vi "Initalize (seq）(SubVI).vi"(10 "字符串":string, 11 "队列输入":refnum<queue>) -> ()   [LabVIEW 2019, in "Take Seq.lvlib"]
uses:
  Take Seq.lvlib
  config.ctl
  Instrument.ctl
  lib/QDInstrument.dll
  SubVI.lvlib
panel:
  # "(真是通道1，假是通道2)"
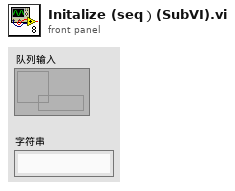
[diagram p1: front panel]
types:
  T1 = typedef "config.ctl" = cluster{"initialize":string, "6221":cluster{"6221 Resource":refnum<visa-resource-name>, "Delta status":bool}, "7001":cluster{"Ch":bool}, "SR830+6221":cluster{"source":u16, "阻抗":dbl, "量程入 4":i32, "量程入 3":i32, "量程入 2":i32, "量程入 1":i32, "电流":dbl, "SR830 2":bool, "SR830 3":bool, "SR830 4":bool, "SR830 1":bool, "VISA 1":refnum<visa-resource-name>, "VISA 2":refnum<visa-resource-name>, "VISA 3":refnum<visa-resource-name>, "VISA 4":refnum<visa-resource-name>, "量程":enum16{"量程每次测量会判定", "量程不变为设定值"}}, "2400":cluster{"2400":bool, "VISA":refnum<visa-resource-name>}, "ch":cluster{"ch str":string, "ch1":bool, "ch2":bool, "布尔":bool}, "error":bool, "数据文件路径":path, "log":cluster{"log路径":path, "log interval":dbl}, "Instrument":T2}
  T2 = typedef "Instrument.ctl" = cluster{"335 Resource":refnum<visa-resource-name>, "Input (0:A)":u16, "Instrument Type":i32, "quantum design":refnum<k24>, "Heater Output (1:1)":u16}
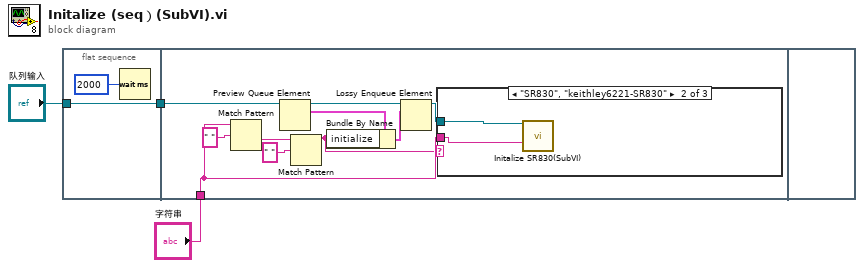
[diagram p0: block diagram]
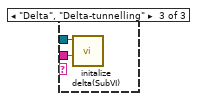
[diagram p3: hidden frame]
diagram:
  n1 = flat-sequence {
    tunnel: "队列输入" -> [w4]
    tunnel: [w4] -> w3
    tunnel: w3 -> [w11]
    tunnel: "字符串" -> [w12]
    frame #0 {
      n2 = Wait (ms)(milliseconds to wait=u32 2000) -> ()  [unwired: 1 out]
    }
    frame #1 {
      n3 = Match Pattern(string=w12, regular expression=" " ("正则表达式")) -> (after substring=w14:string)  [unwired: 1 in, 3 out]
      n4 = Preview Queue Element(queue=w11) -> (queue out=w9:refnum<queue>, element=w8:T1)  [unwired: 2 in, 2 out]
      n5 = Match Pattern(string=w14, regular expression=" " ("正则表达式")) -> (before substring=w6:string)  [unwired: 1 in, 3 out]
      n6 = Bundle By Name(cluster=w8, "initialize"=w6) -> (w10:T1)
      n7 = Lossy Enqueue Element(queue=w9, element=w10) -> (queue out=w7:refnum<queue>)  [unwired: 1 in, 3 out]
      n8 = case shown="\"SR830\", \"keithley6221-SR830\"" w6 {
        tunnel: w12 -> [_ w16 w19]
        tunnel: w7 -> [_ w17 w18]
        frame "假", Default {
        }
        frame "SR830", "keithley6221-SR830" {
          n9 = call "Initalize SR830(SubVI).vi"("队列输入"=w17, "字符串"=w16) -> ()  [unwired: 14 in]
        }
        frame "Delta", "Delta-tunnelling" {
          n10 = call "initalize delta(SubVI).vi"("字符串"=w19, "队列输出"=w18) -> ()  [unwired: 10 in]
        }
      }
    }
    frame #2 {
    }
  }
